vi "Clear Error 1122.vi"(11 "error in":errorcluster) -> (3 "error out":errorcluster)   [LabVIEW 8.6]
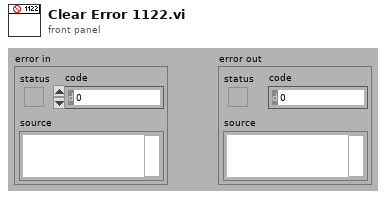
[diagram p1: front panel]
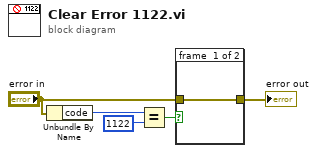
[diagram p0: block diagram]
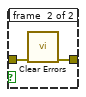
[diagram p2: hidden frame]
diagram:
  n1 = Unbundle By Name("error in") -> ("code"=w1:i32)
  n2 = Equal?(x=w1, y=1122) -> (x = y?=w3:bool)
  n3 = case shown="True" w3 {
    tunnel: "error in" -> [w6 w8]
    tunnel: [w6 w7] -> w5
    frame #0 {
    }
    frame #1 {
      n4 = call <vilib>:"Clear Errors.vi"("error in (no error)"=w8) -> ("error out"=w7:errorcluster)  [unwired: 6 in]
    }
  }
  "error out" <- w5
